vi "hub_geti.vi"(3 "错误输入（无错误）":errorcluster, 4 "输入 1":i32, 5 "VISA资源名称":refnum<visa-resource-name>) -> (0 "错误输出":errorcluster, 1 "数字":i32, 2 "VISA资源名称输出":refnum<visa-resource-name>)   [LabVIEW 2017]
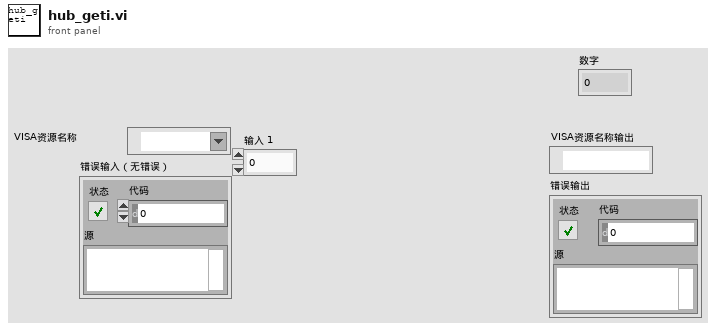
[diagram p1: front panel]
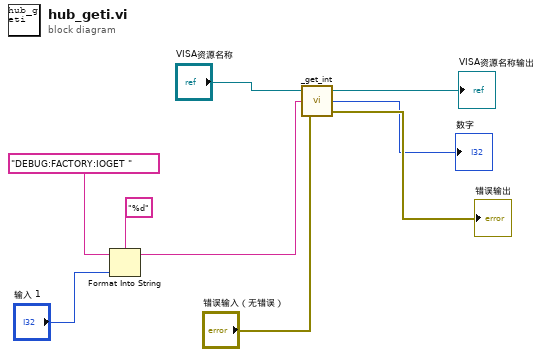
[diagram p0: block diagram]
diagram:
  n1 = Format Into String(format string="%d" ("格式字符串"), initial string="DEBUG:FACTORY:IOGET " ("初始字符串"), "输入 1") -> (resulting string=w3:string)  [unwired: 1 in, 1 out]
  n2 = call "_get_int.vi"("错误输入（无错误）"="错误输入（无错误）", "写入缓冲区"=w3, "VISA资源名称"="VISA资源名称") -> ("错误输出"=→"错误输出":errorcluster, "数字"=→"数字":i32, "VISA资源名称输出"=→"VISA资源名称输出":refnum<visa-resource-name>)
